vi "Omega Get Data.vi"(2 "Point #":i32, 3 "Command String":string, 4 "GPIB Address":refnum<visa-resource-name>) -> (0 "Stop":bool, 1 "Measurement":dbl[](array[numeric]) format="%.2e")   [LabVIEW 2021]
doc: "This VI reads a single reading from an Omega CNi32 temperature controller. The stop boolean is always false. If no reading is obtained a single zero is returned. Adapted from code by Scott Hannahs.\nJonathan Billings, NHMFL-FSU, Jan 2008"
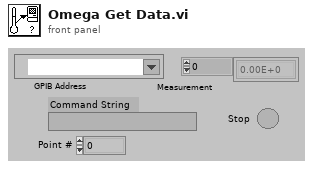
[diagram p1: front panel]
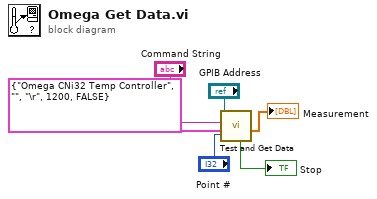
[diagram p0: block diagram]
diagram:
  n1 = call "Test and Get Data.vi"("Point #"="Point #", "Instrument Info"=cluster{string, string, string, u32, bool} {"Omega CNi32 Temp Controller", "", "\r", 1200, FALSE}, "Command String"="Command String", "VISA Sesson"="GPIB Address") -> ("Measurement"=→"Measurement":dbl[], "Stop"=→"Stop":bool)  [unwired: 2 in, 3 out]
